vi "Set LED Status.vi"() -> ()   [LabVIEW 2011]
uses:
  <vilib>/LabVIEW Hacker/LVH-Interface-for-Kinect/Public/Type Defs/LED State.ctl
  <vilib>/LabVIEW Hacker/LVH-Interface-for-Kinect/LVH-Interface-for-Kinect.lvlib
panel:
  in  "Stop Button":bool
  in  "Blink Red-Yellow":bool
  in  "Blink Green":bool
  in  "Yellow":bool
  in  "Red":bool
  in  "Green":bool
  in  "Off":bool
  # "Run this VI\nClick one of the LED State buttons to set the LED.\nClick stop to exit."
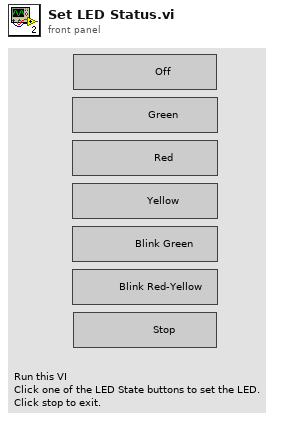
[diagram p1: front panel]
types:
  T1 = typedef "LVH-Interface-for-Kinect.lvlib/LED State.ctl" = enum16{"Off", "Green", "Red", "Yellow", "Blink Green", "Reserved", "Blink Red-Yellow"}
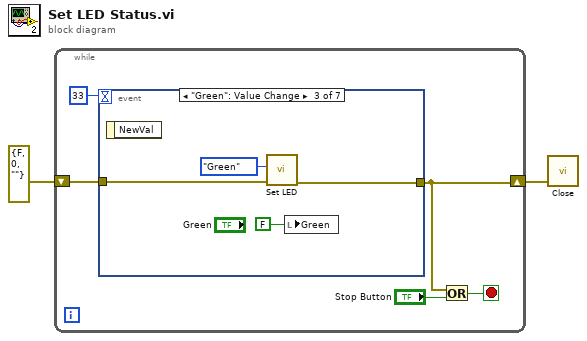
[diagram p0: block diagram]
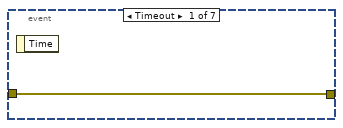
[diagram p2: hidden frame]
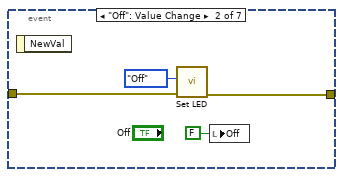
[diagram p3: hidden frame]
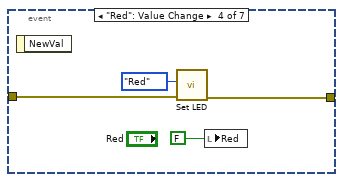
[diagram p4: hidden frame]
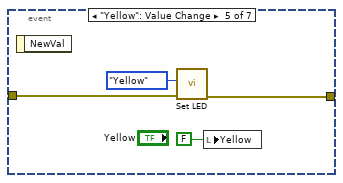
[diagram p5: hidden frame]
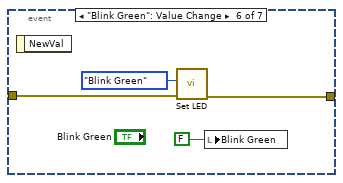
[diagram p6: hidden frame]
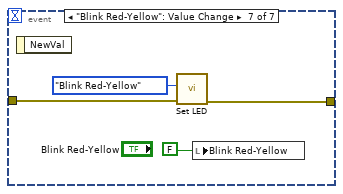
[diagram p7: hidden frame]
diagram:
  n1 = while {
    shift-right: [w3] -> w1
    shift-left: errorcluster {"status"=FALSE, "code"=0, "source"=""} ("Error In") -> [w6]
    stop <- w5 stop-if-true
    n2 = event shown="[2] \"Green\": Value Change" {
      selector: _ -> [_ _ _ _ _ _ _]
      dyn-events: _ -> [_ _ _ _ _ _ _]
      timeout: 33 -> [_ _ _ _ _ _ _]
      tunnel: w6 -> [w8 w11 w15 w19 w23 w27 w31]
      tunnel: [w8 w10 w14 w18 w22 w26 w30] -> w3
      event Timeout {
        n3 = event-data() -> ()  [unwired: 1 in, 1 out]
      }
      event "Off": Value Change {
        n4 = event-data() -> ()  [unwired: 1 in, 1 out]
        n5 = call <vilib>:"Set LED.vi"("Error In"=w11, "LED State"=LED_State."Off") -> ("Error Out"=w10:errorcluster)  [unwired: 9 in]
        n6 = local write "Off"(FALSE ("Off")) -> ()
      }
      event "Green": Value Change {
        n7 = event-data() -> ()  [unwired: 1 in, 1 out]
        n8 = call <vilib>:"Set LED.vi"("Error In"=w15, "LED State"=LED_State."Green") -> ("Error Out"=w14:errorcluster)  [unwired: 9 in]
        n9 = local write "Green"(FALSE ("Off")) -> ()
      }
      event "Red": Value Change {
        n10 = event-data() -> ()  [unwired: 1 in, 1 out]
        n11 = call <vilib>:"Set LED.vi"("Error In"=w19, "LED State"=LED_State."Red") -> ("Error Out"=w18:errorcluster)  [unwired: 9 in]
        n12 = local write "Red"(FALSE ("Off")) -> ()
      }
      event "Yellow": Value Change {
        n13 = event-data() -> ()  [unwired: 1 in, 1 out]
        n14 = call <vilib>:"Set LED.vi"("Error In"=w23, "LED State"=LED_State."Yellow") -> ("Error Out"=w22:errorcluster)  [unwired: 9 in]
        n15 = local write "Yellow"(FALSE ("Off")) -> ()
      }
      event "Blink Green": Value Change {
        n16 = event-data() -> ()  [unwired: 1 in, 1 out]
        n17 = call <vilib>:"Set LED.vi"("Error In"=w27, "LED State"=LED_State."Blink Green") -> ("Error Out"=w26:errorcluster)  [unwired: 9 in]
        n18 = local write "Blink Green"(FALSE ("Off")) -> ()
      }
      event "Blink Red-Yellow": Value Change {
        n19 = event-data() -> ()  [unwired: 1 in, 1 out]
        n20 = call <vilib>:"Set LED.vi"("Error In"=w31, "LED State"=LED_State."Blink Red-Yellow") -> ("Error Out"=w30:errorcluster)  [unwired: 9 in]
        n21 = local write "Blink Red-Yellow"(FALSE ("Off")) -> ()
      }
    }
    n22 = Or(x=w3, y="Stop Button") -> (x .or. y?=w5:bool)
  }
  n23 = call <vilib>:"Close.vi"("Error In"=w1) -> ()  [unwired: 10 in, 1 out]
